vi "Write Loop number.vi"(8 "error in (no error)":errorcluster, 10 "Loop number":i32, 11 "Background Loop Msg in":refnum<class "Background Loop Msg.lvclass">) -> (0 "error out":errorcluster, 3 "Background Loop Msg out":refnum<class "Background Loop Msg.lvclass">)   [LabVIEW 2021, in "Background Loop Msg.lvclass"]
uses:
  Background Loop Msg.lvclass
  Background Loop Msg.lvclass/Background Loop Msg.ctl
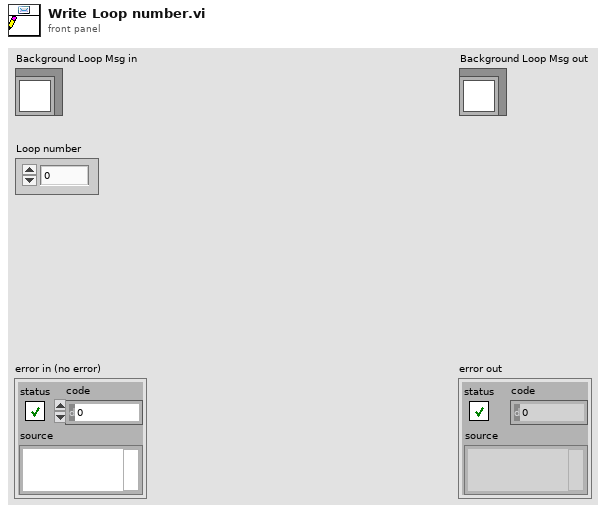
[diagram p1: front panel]
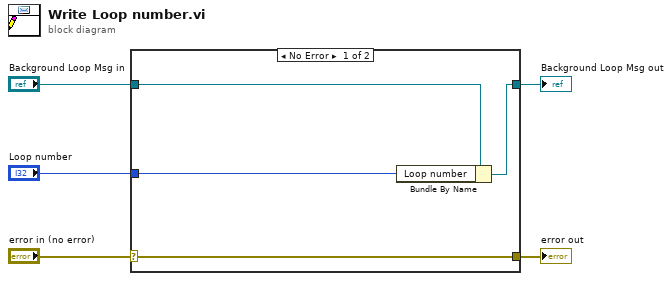
[diagram p0: block diagram]
diagram:
  n1 = case shown="No Error" "error in (no error)" {
    selector: "error in (no error)" -> [w9 w10]
    tunnel: [w9 w10] -> w4
    tunnel: [w7 w11] -> w2
    tunnel: "Background Loop Msg in" -> [w8 w11]
    tunnel: "Loop number" -> [w6 _]
    frame No Error {
      n2 = Bundle By Name(cluster=w8, "Loop number"=w6) -> (w7:refnum<class "Background Loop Msg.lvclass">)
    }
    frame Error {
    }
  }
  "error out" <- w4
  "Background Loop Msg out" <- w2
